vi "oa_FIR Preprocess Filter Param Validation.vi"(6 "fs [Hz]":dbl=1.0, 7 "filter types":T2(ring), 8 "error in (no error)":errorcluster, 10 "ripple specs [dB]":cluster{"pass band":dbl, "stop band":dbl}={"pass band"=0.1, "stop band"=60.0} {"stop band" format="%0.2f"; "pass band" format="%0.2f"}, 11 "freq specs [Hz]":T1={"fpass 1"=0.125, "fstop 1"=0.45, "fpass 2"=0.125, "fstop 2"=0.45} {"fstop 2" format="%0.2f"; "fpass 2" format="%.3f"; "fstop 1" format="%0.2f"; "fpass 1" format="%.3f"}) -> (0 "error out":errorcluster, 2 "dup ripple specs [dB]":cluster{"pass band":dbl, "stop band":dbl}={"pass band"=0.1, "stop band"=60.0} {"stop band" format="%0.2f"; "pass band" format="%0.2f"}, 3 "dup freq specs [Hz]":T1={"fpass 1"=0.125, "fstop 1"=0.45, "fpass 2"=0.125, "fstop 2"=0.45} {"fstop 2" format="%0.2f"; "fpass 2" format="%.3f"; "fstop 1" format="%0.2f"; "fpass 1" format="%.3f"})   [LabVIEW 2017, in "SoundVib_RefDataProcess.lvlib"]
uses:
  <vilib>/addons/Sound and Vibration/Order Analysis/Referece Data Processing/SoundVib_RefDataProcess.lvlib
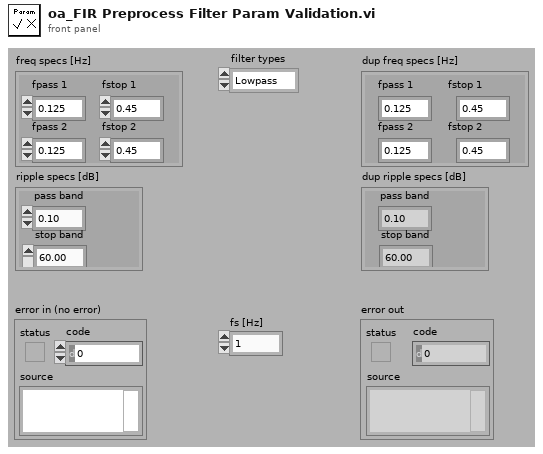
[diagram p1: front panel]
types:
  T1 = cluster{"fpass 1":dbl, "fstop 1":dbl, "fpass 2":dbl, "fstop 2":dbl}
  T2 = enum32{"Lowpass", "Highpass", "Bandpass", "Bandstop"}
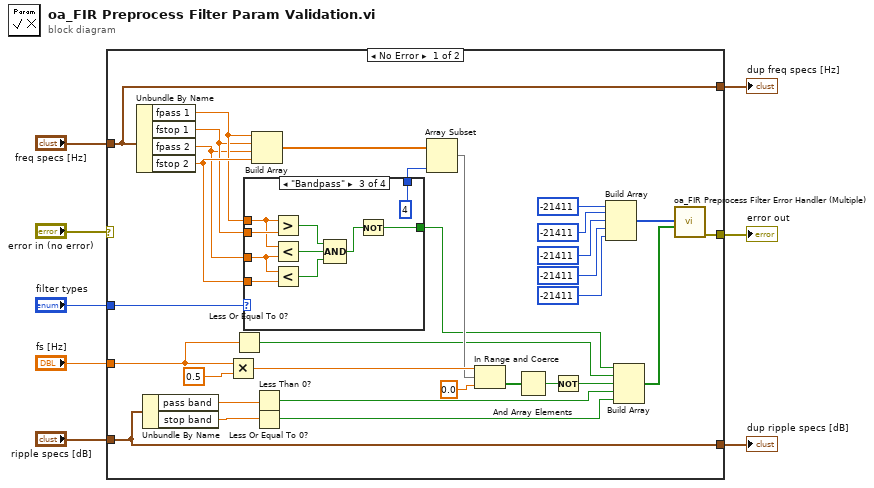
[diagram p0: block diagram]
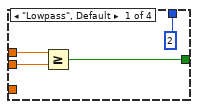
[diagram p2: hidden frame]
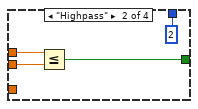
[diagram p3: hidden frame]
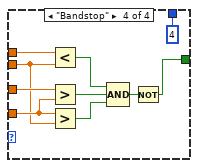
[diagram p4: hidden frame]
diagram:
  n1 = case shown="No Error" "error in (no error)" {
    selector: "error in (no error)" -> [_ w68]
    tunnel: "freq specs [Hz]" -> [w13 _]
    tunnel: "fs [Hz]" -> [w35 _]
    tunnel: "ripple specs [dB]" -> [w12 _]
    tunnel: "filter types" -> [w32 _]
    tunnel: [w16 w68] -> w4
    tunnel: [w13 _] -> w2
    tunnel: [w12 _] -> w1
    frame No Error {
      n2 = Unbundle By Name(w13) -> ("fpass 1"=w29:dbl, "fstop 1"=w28:dbl, "fpass 2"=w27:dbl, "fstop 2"=w30:dbl)
      n3 = Unbundle By Name(w12) -> ("pass band"=w26:dbl, "stop band"=w25:dbl)
      n4 = Multiply(x=w35, y=0.5) -> (x*y=w38:dbl)
      n5 = Less Or Equal To 0?(x=w35) -> (x <= 0?=w14:bool)
      n6 = case shown="\"Bandpass\"" w32 {
        tunnel: [2 2 4 4] -> w31
        tunnel: w30 -> [_ _ w54 w64]
        tunnel: w29 -> [w42 w45 w55 w66]
        tunnel: w28 -> [w41 w44 w56 w63]
        tunnel: w27 -> [_ _ w49 w65]
        tunnel: [w40 w46 w48 w58] -> w10
        frame "Lowpass", Default {
          n7 = Greater Or Equal?(x=w42, y=w41) -> (x >= y?=w40:bool)
        }
        frame "Highpass" {
          n8 = Less Or Equal?(x=w45, y=w44) -> (x <= y?=w46:bool)
        }
        frame "Bandpass" {
          n9 = Greater?(x=w55, y=w56) -> (0:w53:bool)
          n10 = Less?(x=w55, y=w49) -> (x < y?=w52:bool)
          n11 = Less?(x=w49, y=w54) -> (x < y?=w51:bool)
          n12 = Compound Arithmetic op=AND(w53, w52, w51) -> (w50:bool)
          n13 = Not(x=w50) -> (.not. x?=w48:bool)
        }
        frame "Bandstop" {
          n14 = Less?(x=w66, y=w63) -> (x < y?=w62:bool)
          n15 = Greater?(x=w65, y=w64) -> (0:w61:bool)
          n16 = Greater?(x=w64, y=w63) -> (0:w60:bool)
          n17 = Compound Arithmetic op=AND(w62, w61, w60) -> (w59:bool)
          n18 = Not(x=w59) -> (.not. x?=w58:bool)
        }
      }
      n19 = Build Array(w29, w28, w27, w30) -> (w36:dbl[])
      n20 = Less Than 0?(x=w26) -> (x < 0?=w24:bool)
      n21 = Less Or Equal To 0?(x=w25) -> (x <= 0?=w23:bool)
      n22 = Array Subset(array=w36, length=w31) -> (w33:dbl[])  [unwired: 1 in]
      n23 = In Range and Coerce(upper limit=w38, x=w33, lower limit=0.0) -> (In Range?=w34:bool[])  [unwired: 1 out]
      n24 = And Array Elements(Boolean array=w34) -> (logical AND=w15:bool)
      n25 = Not(x=w15) -> (.not. x?=w11:bool)
      n26 = Build Array(-21411, -21411, -21411, -21411, -21411) -> (w17:i32[])
      n27 = Build Array(w10, w14, w11, w24, w23) -> (w9:bool[])
      n28 = call <vilib>:"oa_FIR Preprocess Filter Error Handler (Multiple).vi"("condition failed?"=w9, "error sources"=w17) -> ("error out"=w16:errorcluster)  [unwired: 9 in]
    }
    frame Error {
    }
  }
  "dup freq specs [Hz]" <- w2
  "dup ripple specs [dB]" <- w1
  "error out" <- w4
